vi "Launch Nested Actors.vi"(8 "error in (no error)":errorcluster, 11 "CO2 Actor in":refnum<class "CO2 Actor.lvclass">) -> (0 "error out":errorcluster, 3 "CO2 Actor out":refnum<class "CO2 Actor.lvclass">)   [LabVIEW 2015, in "cRIO-Carbondioxide.lvlib" / "CO2-Actor.lvlib" / "CO2 Actor.lvclass"]
uses:
  CO2 Actor.lvclass
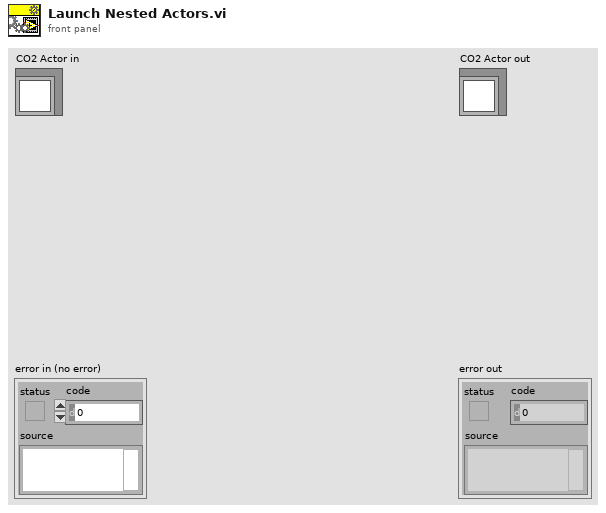
[diagram p1: front panel]
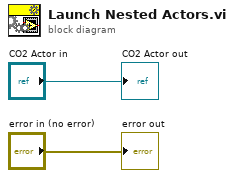
[diagram p0: block diagram]
diagram:
  "error out" <- "error in (no error)"
  "CO2 Actor out" <- "CO2 Actor in"
